vi "wait.vi"(8 "Ts (ms)":u32, 11 "Qube":refnum<class "Qube.lvclass">) -> (0 "dt":dbl format="%.2f", 3 "Qube":refnum<class "Qube.lvclass">)   [LabVIEW 2017, in "Qube.lvclass"]
uses:
  Qube.lvclass
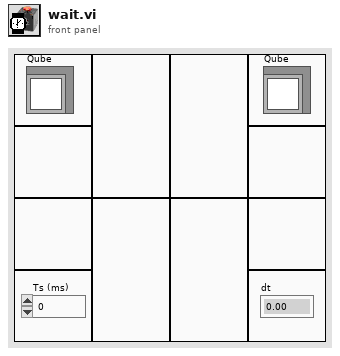
[diagram p1: front panel]
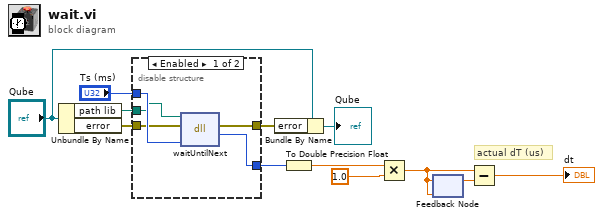
[diagram p0: block diagram]
diagram:
  # "actual dT (us)"
  n1 = Unbundle By Name("Qube") -> ("path lib"=w10:path, "error"=w2:errorcluster)
  n2 = disable-structure shown="Enabled" {
    disable-tunnel: w10 -> [w16 _]
    disable-tunnel: w2 -> [w15 _]
    disable-tunnel: [w14 _] -> w9
    disable-tunnel: [w13 _] -> w1
    disable-tunnel: "Ts (ms)" -> [w17 _]
    frame Enabled {
      n3 = dll-call lib="Users/philippe/Desktop/cpp/LibLoader/libLoader.so" fn="waitUntilNext"(path in=w16, error in=w15, "Ts (ms)"=w17) -> (error out=w14:errorcluster, "time (us)"=w13:i32)  [unwired: 2 in, 1 out]
    }
    frame Disabled {
    }
  }
  n4 = Bundle By Name(cluster="Qube", "error"=w9) -> (→"Qube":refnum<class "Qube.lvclass">)
  n5 = To Double Precision Float(number=w1) -> (double precision float=w5:dbl)
  n6 = Multiply(x=w5, y=1.0) -> (x*y=w4:dbl)
  n7 = feedback #1(w4) -> (w8:dbl)
  n8 = feedback-in #1(w4) -> ()
  n9 = Subtract(x=w4, y=w8) -> (x-y=→"dt":dbl)
